vi "SVT Motors.vi"   [LabVIEW 2017, in "SoundVib_MachineCharacteristic.lvlib"]
doc: "Calculates characteristic frequencies or orders of motors. You must manually select the polymorphic instance you want to use."
uses:
  <vilib>/addons/Sound and Vibration/svt_Machine Characteristic/SoundVib_MachineCharacteristic.lvlib
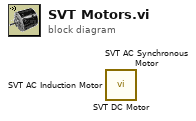
[diagram p0: block diagram]
diagram:
  n1 = call <vilib>:"SVT DC Motor.vi"() -> ()  [unwired: 13 in, 3 out]
  n2 = call <vilib>:"SVT AC Synchronous Motor.vi"() -> ()  [unwired: 13 in, 3 out]
  n3 = call <vilib>:"SVT AC Induction Motor.vi"() -> ()  [unwired: 11 in, 5 out]
